vi "input.vi"(8 "error in":errorcluster, 10 "data table in":T1, 11 "OPC UA runtime in":refnum<class "OPC UA Client runtime.lvclass">) -> (0 "error out":errorcluster, 2 "data table out":T1, 3 "OPC UA runtime out":refnum<class "OPC UA Client runtime.lvclass">)   [LabVIEW 2013, in "OPC UA Client runtime.lvclass"]
doc: "Provides an interface for reading data from a module at runtime. While this interface performs no operations, a child should provide an override which may read from any open sessions, references, or interfaces."
uses:
  OPC UA Client runtime.lvclass
  <vilib>/NI/Tag Bus/table/data table.ctl
  OPC UA Client runtime.lvclass/OPC UA Client runtime.ctl
  <vilib>/NI/Tag Bus/table/data polymorphs/write one/write Boolean.vi
  <vilib>/NI/Tag Bus/table/data polymorphs/write one/write I8.vi
  <vilib>/NI/Tag Bus/table/data polymorphs/write one/write U8.vi
  <vilib>/NI/Tag Bus/table/data polymorphs/write one/write I16.vi
  <vilib>/NI/Tag Bus/table/data polymorphs/write one/write U16.vi
  <vilib>/NI/Tag Bus/table/data polymorphs/write one/write I32.vi
  <vilib>/NI/Tag Bus/table/data polymorphs/write one/write U32.vi
  <vilib>/NI/Tag Bus/table/data polymorphs/write one/write I64.vi
  <vilib>/NI/Tag Bus/table/data polymorphs/write one/write U64.vi
  <vilib>/NI/Tag Bus/table/data polymorphs/write one/write Single.vi
  <vilib>/NI/Tag Bus/table/data polymorphs/write one/write Double.vi
  <vilib>/NI/Tag Bus/table/data polymorphs/write one/write String.vi
  <vilib>/NI/Tag Bus/table/data polymorphs/write one/write Array of Boolean.vi
  <vilib>/NI/Tag Bus/table/data polymorphs/write one/write Array of I8.vi
  <vilib>/NI/Tag Bus/table/data polymorphs/write one/write Array of U8.vi
  <vilib>/NI/Tag Bus/table/data polymorphs/write one/write Array of I16.vi
  <vilib>/NI/Tag Bus/table/data polymorphs/write one/write Array of U16.vi
  <vilib>/NI/Tag Bus/table/data polymorphs/write one/write Array of I32.vi
  <vilib>/NI/Tag Bus/table/data polymorphs/write one/write Array of U32.vi
  <vilib>/NI/Tag Bus/table/data polymorphs/write one/write Array of I64.vi
  <vilib>/NI/Tag Bus/table/data polymorphs/write one/write Array of U64.vi
  <vilib>/NI/Tag Bus/table/data polymorphs/write one/write Array of Single.vi
  <vilib>/NI/Tag Bus/table/data polymorphs/write one/write Array of Double.vi
  <vilib>/NI/Tag Bus/table/data polymorphs/write one/write Array of String.vi
  <vilib>/OPCUA/client/Read Bool.vi
  <vilib>/OPCUA/client/Read SByte.vi
  <vilib>/OPCUA/client/Read Byte.vi
  <vilib>/OPCUA/client/Read Int16.vi
  <vilib>/OPCUA/client/Read UInt16.vi
  <vilib>/OPCUA/client/Read Int32.vi
  <vilib>/OPCUA/client/Read UInt32.vi
  <vilib>/OPCUA/client/Read Int64.vi
  <vilib>/OPCUA/client/Read UInt64.vi
  <vilib>/OPCUA/client/Read Float.vi
  <vilib>/OPCUA/client/Read Double.vi
  <vilib>/OPCUA/client/Read String.vi
  <vilib>/OPCUA/client/Read DateTime.vi
  <vilib>/OPCUA/client/Read ByteString.vi
  <vilib>/OPCUA/client/Read Bool Array.vi
  <vilib>/OPCUA/client/Read SByte Array.vi
  <vilib>/OPCUA/client/Read Byte Array.vi
  <vilib>/OPCUA/client/Read Int16 Array.vi
  <vilib>/OPCUA/client/Read UInt16 Array.vi
  <vilib>/OPCUA/client/Read Int32 Array.vi
  <vilib>/OPCUA/client/Read UInt32 Array.vi
  <vilib>/OPCUA/client/Read Int64 Array.vi
  <vilib>/OPCUA/client/Read UInt64 Array.vi
  <vilib>/OPCUA/client/Read Float Array.vi
  <vilib>/OPCUA/client/Read Double Array.vi
  <vilib>/OPCUA/client/Read String Array.vi
  <vilib>/OPCUA/client/Read DateTime Array.vi
  <vilib>/OPCUA/client/Read ByteString Array.vi
  <vilib>/Utility/error.llb/Error Cluster From Error Code.vi
  <vilib>/ErrorRing/Error Ring.xnode
  <vilib>/NI/Tag Bus/table/data table.lvlib
  <vilib>/opcua/NI OPC UA Client.lvlib
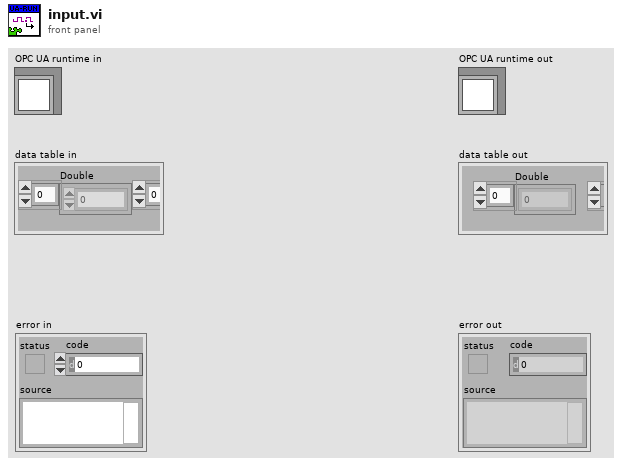
[diagram p1: front panel]
types:
  T1 = typedef "tag bus.lvlib/data table.lvlib/data table.ctl" = cluster{"Double":dbl[], "Single":sgl[], "I64":i64[], "I32":i32[], "I16":i16[], "I8":i8[], "U64":u64[], "U32":u32[], "U16":u16[], "U8":u8[], "Boolean":bool[], "String":string[], "Array of Double":cluster{"DBL Array":dbl[]}[], "Array of Single":cluster{"SGL Array":sgl[]}[], "Array of I64":cluster{"I64 Array":i64[]}[], "Array of I32":cluster{"I32 Array":i32[]}[], "Array of I16":cluster{"I16 Array":i16[]}[], "Array of I8":cluster{"I8 Array":i8[]}[], "Array of U64":cluster{"U64 Array":u64[]}[], "Array of U32":cluster{"U32 Array":u32[]}[], "Array of U16":cluster{"U16 Array":u16[]}[], "Array of U8":cluster{"U8 Array":u8[]}[], "Array of Boolean":cluster{"Boolean Array":bool[]}[], "Array of String":cluster{"String Array":string[]}[]}
  T2 = typedef "tag bus.lvlib/tag descriptor.lvclass/Data Type.ctl" = enum16{"Double", "Single", "I64", "I32", "I16", "I8", "U64", "U32", "U16", "U8", "Boolean", "String", "Array of Double", "Array of Single", "Array of I64", "Array of I32", "Array of I16", "Array of I8", "Array of U64", "Array of U32", "Array of U16", "Array of U8", "Array of Boolean", "Array of String"}
  T3 = typedef "OPC UA Client configuration.lvclass/OPC UA Data Type.ctl" = u16
  T4 = cluster{"DCAF Data Type":T2, "Index":i32, "Node Path":string, "OPC UA Data Type":T3}[]
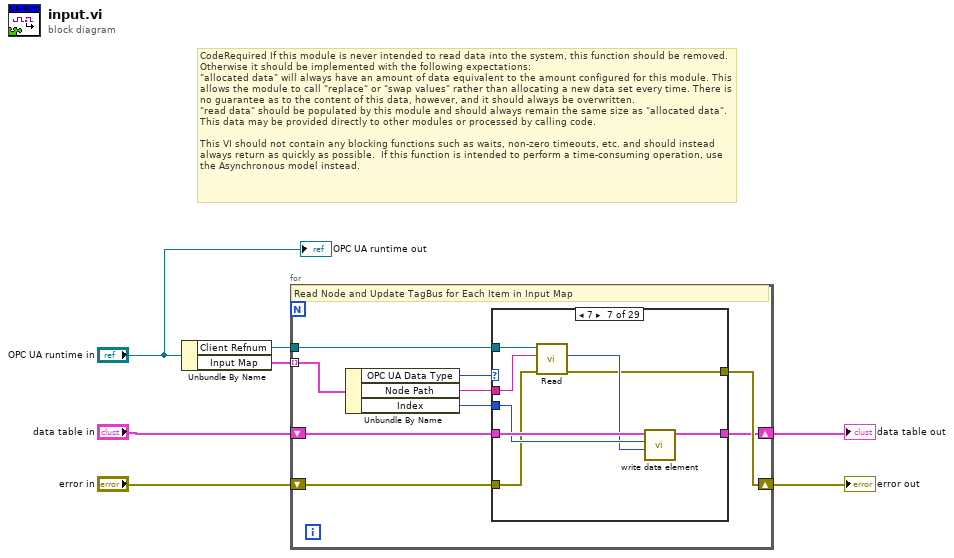
[diagram p0: block diagram]
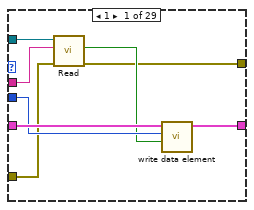
[diagram p2: hidden frame]
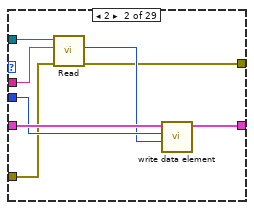
[diagram p3: hidden frame]
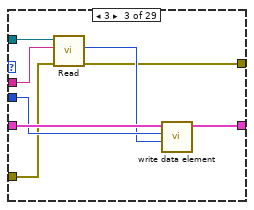
[diagram p4: hidden frame]
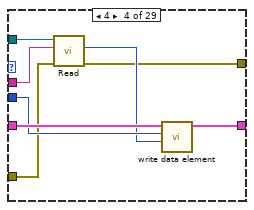
[diagram p5: hidden frame]
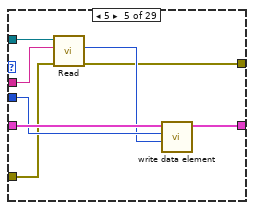
[diagram p6: hidden frame]
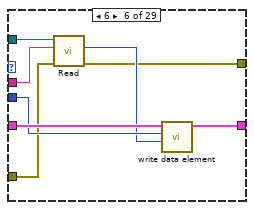
[diagram p7: hidden frame]
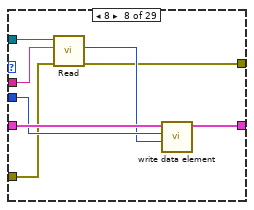
[diagram p8: hidden frame]
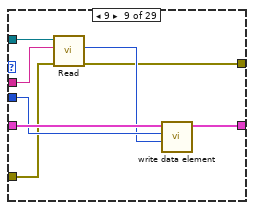
[diagram p9: hidden frame]
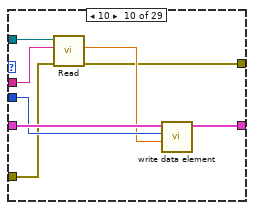
[diagram p10: hidden frame]
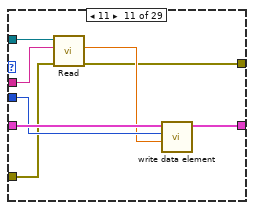
[diagram p11: hidden frame]
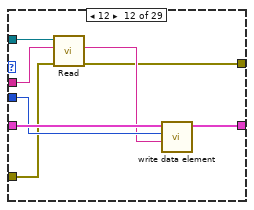
[diagram p12: hidden frame]
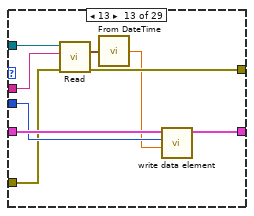
[diagram p13: hidden frame]
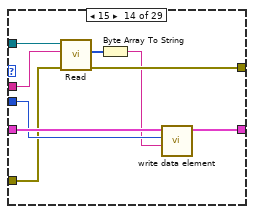
[diagram p14: hidden frame]
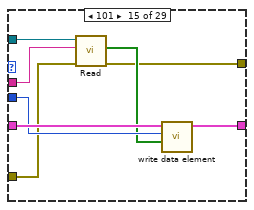
[diagram p15: hidden frame]
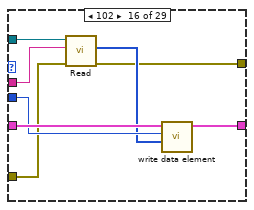
[diagram p16: hidden frame]
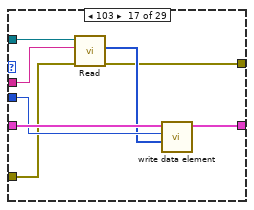
[diagram p17: hidden frame]
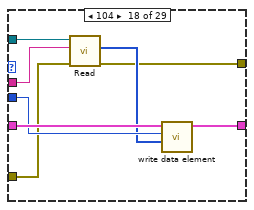
[diagram p18: hidden frame]
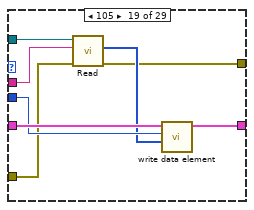
[diagram p19: hidden frame]
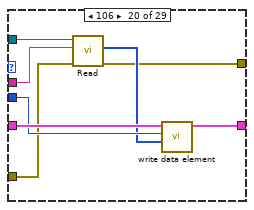
[diagram p20: hidden frame]
diagram:
  # "CodeRequired If this module is never intended to read data into the system, this function should be removed. Otherwise it should be implemented with the following expectations:\n\"allocated data\" will always have an amount of data equivalent to the amount configured for this module. This allows the module to call \"replace\" or \"swap values\" rather than allocating a new data set every time. There is no guarantee as to the content of this data, however, and it should always be overwritten.\n\"read data\" should be populated by this module and should always remain the same size as \"allocated data\". This data may be provided directly to other modules or processed by calling code.\n\nThis VI should not contain any blocking functions such as waits, non-zero timeouts, etc. and should instead always return as quickly as possible.  If this function is intended to perform a time-consuming operation, use the Asynchronous model instead."
  n1 = Unbundle By Name("OPC UA runtime in") -> ("Client Refnum"=w2:refnum<k21>, "Input Map"=w1:T4)
  n2 = for {
    tunnel: w2 -> [w12]
    tunnel: w1 -> [w16] mode=indexing
    shift-right: [w9] -> w3
    shift-left: "error in" -> [w10]
    shift-right: [w8] -> w4
    shift-left: "data table in" -> [w11]
    # "Read Node and Update TagBus for Each Item in Input Map"
    n3 = Unbundle By Name(w16) -> ("OPC UA Data Type"=w15:T3, "Node Path"=w14:string, "Index"=w13:i32)
    n4 = case shown="7" w15 {
      tunnel: w14 -> [w23 w31 w39 w47 w55 w63 w71 w79 w87 w95 w103 w111 w120 w129 w137 w145 w153 w161 w169 w177 w185 w193 w201 w209 w217 w225 w234 w243 _]
      tunnel: w13 -> [w21 w29 w37 w45 w53 w61 w69 w77 w85 w93 w101 w109 w118 w127 w135 w143 w151 w159 w167 w175 w183 w191 w199 w207 w215 w223 w232 w241 _]
      tunnel: w12 -> [w24 w32 w40 w48 w56 w64 w72 w80 w88 w96 w104 w112 w121 w130 w138 w146 w154 w162 w170 w178 w186 w194 w202 w210 w218 w226 w235 w244 _]
      tunnel: w11 -> [w22 w30 w38 w46 w54 w62 w70 w78 w86 w94 w102 w110 w119 w128 w136 w144 w152 w160 w168 w176 w184 w192 w200 w208 w216 w224 w233 w242 w247]
      tunnel: w10 -> [w19 w27 w35 w43 w51 w59 w67 w75 w83 w91 w99 w107 w117 w126 w133 w141 w149 w157 w165 w173 w181 w189 w197 w205 w213 w221 w231 w240 _]
      tunnel: [w18 w26 w34 w42 w50 w58 w66 w74 w82 w90 w98 w106 w116 w125 w132 w140 w148 w156 w164 w172 w180 w188 w196 w204 w212 w220 w230 w239 w248] -> w9
      tunnel: [w17 w25 w33 w41 w49 w57 w65 w73 w81 w89 w97 w105 w115 w124 w131 w139 w147 w155 w163 w171 w179 w187 w195 w203 w211 w219 w229 w238 w247] -> w8
      frame 1 {
        n5 = call-poly <vilib>:"Read.vi"("error in (no error)"=w19, "node path"=w23, "OPC UA client refnum in"=w24) -> ("error out"=w18:errorcluster, "value"=w20:bool)  [unwired: 4 in, 3 out]
        n6 = call-poly <vilib>:"write data element.vi"("value"=w20, "index"=w21, "data table in"=w22) -> ("data table out"=w17:T1)  [unwired: 8 in]
      }
      frame 2 {
        n7 = call-poly <vilib>:"Read.vi"("error in (no error)"=w27, "node path"=w31, "OPC UA client refnum in"=w32) -> ("error out"=w26:errorcluster, "value"=w28:i8)  [unwired: 4 in, 3 out]
        n8 = call-poly <vilib>:"write data element.vi"("value"=w28, "index"=w29, "data table in"=w30) -> ("data table out"=w25:T1)  [unwired: 8 in]
      }
      frame 3 {
        n9 = call-poly <vilib>:"Read.vi"("error in (no error)"=w35, "node path"=w39, "OPC UA client refnum in"=w40) -> ("error out"=w34:errorcluster, "value"=w36:u8)  [unwired: 4 in, 3 out]
        n10 = call-poly <vilib>:"write data element.vi"("value"=w36, "index"=w37, "data table in"=w38) -> ("data table out"=w33:T1)  [unwired: 8 in]
      }
      frame 4 {
        n11 = call-poly <vilib>:"Read.vi"("error in (no error)"=w43, "node path"=w47, "OPC UA client refnum in"=w48) -> ("error out"=w42:errorcluster, "value"=w44:i16)  [unwired: 4 in, 3 out]
        n12 = call-poly <vilib>:"write data element.vi"("value"=w44, "index"=w45, "data table in"=w46) -> ("data table out"=w41:T1)  [unwired: 8 in]
      }
      frame 5 {
        n13 = call-poly <vilib>:"Read.vi"("error in (no error)"=w51, "node path"=w55, "OPC UA client refnum in"=w56) -> ("error out"=w50:errorcluster, "value"=w52:u16)  [unwired: 4 in, 3 out]
        n14 = call-poly <vilib>:"write data element.vi"("value"=w52, "index"=w53, "data table in"=w54) -> ("data table out"=w49:T1)  [unwired: 8 in]
      }
      frame 6 {
        n15 = call-poly <vilib>:"Read.vi"("error in (no error)"=w59, "node path"=w63, "OPC UA client refnum in"=w64) -> ("error out"=w58:errorcluster, "value"=w60:i32)  [unwired: 4 in, 3 out]
        n16 = call-poly <vilib>:"write data element.vi"("value"=w60, "index"=w61, "data table in"=w62) -> ("data table out"=w57:T1)  [unwired: 8 in]
      }
      frame 7 {
        n17 = call-poly <vilib>:"Read.vi"("error in (no error)"=w67, "node path"=w71, "OPC UA client refnum in"=w72) -> ("error out"=w66:errorcluster, "value"=w68:u32)  [unwired: 4 in, 3 out]
        n18 = call-poly <vilib>:"write data element.vi"("value"=w68, "index"=w69, "data table in"=w70) -> ("data table out"=w65:T1)  [unwired: 8 in]
      }
      frame 8 {
        n19 = call-poly <vilib>:"Read.vi"("error in (no error)"=w75, "node path"=w79, "OPC UA client refnum in"=w80) -> ("error out"=w74:errorcluster, "value"=w76:i64)  [unwired: 4 in, 3 out]
        n20 = call-poly <vilib>:"write data element.vi"("value"=w76, "index"=w77, "data table in"=w78) -> ("data table out"=w73:T1)  [unwired: 8 in]
      }
      frame 9 {
        n21 = call-poly <vilib>:"Read.vi"("error in (no error)"=w83, "node path"=w87, "OPC UA client refnum in"=w88) -> ("error out"=w82:errorcluster, "value"=w84:u64)  [unwired: 4 in, 3 out]
        n22 = call-poly <vilib>:"write data element.vi"("value"=w84, "index"=w85, "data table in"=w86) -> ("data table out"=w81:T1)  [unwired: 8 in]
      }
      frame 10 {
        n23 = call-poly <vilib>:"Read.vi"("error in (no error)"=w91, "node path"=w95, "OPC UA client refnum in"=w96) -> ("error out"=w90:errorcluster, "value"=w92:sgl)  [unwired: 4 in, 3 out]
        n24 = call-poly <vilib>:"write data element.vi"("value"=w92, "index"=w93, "data table in"=w94) -> ("data table out"=w89:T1)  [unwired: 8 in]
      }
      frame 11 {
        n25 = call-poly <vilib>:"Read.vi"("error in (no error)"=w99, "node path"=w103, "OPC UA client refnum in"=w104) -> ("error out"=w98:errorcluster, "value"=w100:dbl)  [unwired: 4 in, 3 out]
        n26 = call-poly <vilib>:"write data element.vi"("value"=w100, "index"=w101, "data table in"=w102) -> ("data table out"=w97:T1)  [unwired: 8 in]
      }
      frame 12 {
        n27 = call-poly <vilib>:"Read.vi"("error in (no error)"=w107, "node path"=w111, "OPC UA client refnum in"=w112) -> ("error out"=w106:errorcluster, "value"=w108:string)  [unwired: 4 in, 3 out]
        n28 = call-poly <vilib>:"write data element.vi"("value"=w108, "index"=w109, "data table in"=w110) -> ("data table out"=w105:T1)  [unwired: 8 in]
      }
      frame 13 {
        n29 = call-poly <vilib>:"Read.vi"("error in (no error)"=w117, "node path"=w120, "OPC UA client refnum in"=w121) -> ("error out"=w116:errorcluster, "value"=w114:timestamp)  [unwired: 4 in, 3 out]
        n30 = call "From DateTime.vi"("DateTime"=w114) -> ("Formatted DateTime"=w113:dbl)
        n31 = call-poly <vilib>:"write data element.vi"("value"=w113, "index"=w118, "data table in"=w119) -> ("data table out"=w115:T1)  [unwired: 8 in]
      }
      frame 15 {
        n32 = call-poly <vilib>:"Read.vi"("error in (no error)"=w126, "node path"=w129, "OPC UA client refnum in"=w130) -> ("error out"=w125:errorcluster, "value"=w123:u8[])  [unwired: 4 in, 3 out]
        n33 = Byte Array To String(unsigned byte array=w123) -> (string=w122:string)
        n34 = call-poly <vilib>:"write data element.vi"("value"=w122, "index"=w127, "data table in"=w128) -> ("data table out"=w124:T1)  [unwired: 8 in]
      }
      frame 101 {
        n35 = call-poly <vilib>:"Read.vi"("error in (no error)"=w133, "node path"=w137, "OPC UA client refnum in"=w138) -> ("error out"=w132:errorcluster, "value"=w134:bool[])  [unwired: 4 in, 3 out]
        n36 = call-poly <vilib>:"write data element.vi"("value"=w134, "index"=w135, "data table in"=w136) -> ("data table out"=w131:T1)  [unwired: 8 in]
      }
      frame 102 {
        n37 = call-poly <vilib>:"Read.vi"("error in (no error)"=w141, "node path"=w145, "OPC UA client refnum in"=w146) -> ("error out"=w140:errorcluster, "value"=w142:i8[])  [unwired: 4 in, 3 out]
        n38 = call-poly <vilib>:"write data element.vi"("value"=w142, "index"=w143, "data table in"=w144) -> ("data table out"=w139:T1)  [unwired: 8 in]
      }
      frame 103 {
        n39 = call-poly <vilib>:"Read.vi"("error in (no error)"=w149, "node path"=w153, "OPC UA client refnum in"=w154) -> ("error out"=w148:errorcluster, "value"=w150:u8[])  [unwired: 4 in, 3 out]
        n40 = call-poly <vilib>:"write data element.vi"("value"=w150, "index"=w151, "data table in"=w152) -> ("data table out"=w147:T1)  [unwired: 8 in]
      }
      frame 104 {
        n41 = call-poly <vilib>:"Read.vi"("error in (no error)"=w157, "node path"=w161, "OPC UA client refnum in"=w162) -> ("error out"=w156:errorcluster, "value"=w158:i16[])  [unwired: 4 in, 3 out]
        n42 = call-poly <vilib>:"write data element.vi"("value"=w158, "index"=w159, "data table in"=w160) -> ("data table out"=w155:T1)  [unwired: 8 in]
      }
      frame 105 {
        n43 = call-poly <vilib>:"Read.vi"("error in (no error)"=w165, "node path"=w169, "OPC UA client refnum in"=w170) -> ("error out"=w164:errorcluster, "value"=w166:u16[])  [unwired: 4 in, 3 out]
        n44 = call-poly <vilib>:"write data element.vi"("value"=w166, "index"=w167, "data table in"=w168) -> ("data table out"=w163:T1)  [unwired: 8 in]
      }
      frame 106 {
        n45 = call-poly <vilib>:"Read.vi"("error in (no error)"=w173, "node path"=w177, "OPC UA client refnum in"=w178) -> ("error out"=w172:errorcluster, "value"=w174:i32[])  [unwired: 4 in, 3 out]
        n46 = call-poly <vilib>:"write data element.vi"("value"=w174, "index"=w175, "data table in"=w176) -> ("data table out"=w171:T1)  [unwired: 8 in]
      }
      frame 107 {
        n47 = call-poly <vilib>:"Read.vi"("error in (no error)"=w181, "node path"=w185, "OPC UA client refnum in"=w186) -> ("error out"=w180:errorcluster, "value"=w182:u32[])  [unwired: 4 in, 3 out]
        n48 = call-poly <vilib>:"write data element.vi"("value"=w182, "index"=w183, "data table in"=w184) -> ("data table out"=w179:T1)  [unwired: 8 in]
      }
      frame 108 {
        n49 = call-poly <vilib>:"Read.vi"("error in (no error)"=w189, "node path"=w193, "OPC UA client refnum in"=w194) -> ("error out"=w188:errorcluster, "value"=w190:i64[])  [unwired: 4 in, 3 out]
        n50 = call-poly <vilib>:"write data element.vi"("value"=w190, "index"=w191, "data table in"=w192) -> ("data table out"=w187:T1)  [unwired: 8 in]
      }
      frame 109 {
        n51 = call-poly <vilib>:"Read.vi"("error in (no error)"=w197, "node path"=w201, "OPC UA client refnum in"=w202) -> ("error out"=w196:errorcluster, "value"=w198:u64[])  [unwired: 4 in, 3 out]
        n52 = call-poly <vilib>:"write data element.vi"("value"=w198, "index"=w199, "data table in"=w200) -> ("data table out"=w195:T1)  [unwired: 8 in]
      }
      frame 110 {
        n53 = call-poly <vilib>:"Read.vi"("error in (no error)"=w205, "node path"=w209, "OPC UA client refnum in"=w210) -> ("error out"=w204:errorcluster, "value"=w206:sgl[])  [unwired: 4 in, 3 out]
        n54 = call-poly <vilib>:"write data element.vi"("value"=w206, "index"=w207, "data table in"=w208) -> ("data table out"=w203:T1)  [unwired: 8 in]
      }
      frame 111 {
        n55 = call-poly <vilib>:"Read.vi"("error in (no error)"=w213, "node path"=w217, "OPC UA client refnum in"=w218) -> ("error out"=w212:errorcluster, "value"=w214:dbl[])  [unwired: 4 in, 3 out]
        n56 = call-poly <vilib>:"write data element.vi"("value"=w214, "index"=w215, "data table in"=w216) -> ("data table out"=w211:T1)  [unwired: 8 in]
      }
      frame 112 {
        n57 = call-poly <vilib>:"Read.vi"("error in (no error)"=w221, "node path"=w225, "OPC UA client refnum in"=w226) -> ("error out"=w220:errorcluster, "value"=w222:string[])  [unwired: 4 in, 3 out]
        n58 = call-poly <vilib>:"write data element.vi"("value"=w222, "index"=w223, "data table in"=w224) -> ("data table out"=w219:T1)  [unwired: 8 in]
      }
      frame 113 {
        n59 = call-poly <vilib>:"Read.vi"("error in (no error)"=w231, "node path"=w234, "OPC UA client refnum in"=w235) -> ("error out"=w230:errorcluster, "value"=w228:timestamp[])  [unwired: 4 in, 3 out]
        n60 = call "From DateTime Array.vi"("DateTime Array"=w228) -> ("Formatted DateTime Array"=w227:dbl[])
        n61 = call-poly <vilib>:"write data element.vi"("value"=w227, "index"=w232, "data table in"=w233) -> ("data table out"=w229:T1)  [unwired: 8 in]
      }
      frame 115 {
        n62 = call-poly <vilib>:"Read.vi"("error in (no error)"=w240, "node path"=w243, "OPC UA client refnum in"=w244) -> ("error out"=w239:errorcluster, "value"=w237:u8[][])  [unwired: 4 in, 3 out]
        n63 = for {
          tunnel: w237 -> [w246] mode=indexing
          tunnel: [w245] -> w236 mode=indexing
          n64 = Byte Array To String(unsigned byte array=w246) -> (string=w245:string)
        }
        n65 = call-poly <vilib>:"write data element.vi"("value"=w236, "index"=w241, "data table in"=w242) -> ("data table out"=w238:T1)  [unwired: 8 in]
      }
      frame 0, Default {
        # "invalid data type, throw error"
        n66 = xnode "Error Ring"() -> ("error out"=w248:errorcluster)
      }
    }
  }
  "error out" <- w3
  "data table out" <- w4
  "OPC UA runtime out" <- "OPC UA runtime in"
